vi "InfluxDriver.vi"(6 "body":string, 7 "dbwrite":string, 8 "error in (no error)":errorcluster, 9 "authorization":string, 10 "remote port":u16=8086, 11 "InfluxDB Address":string="128.8.27.25") -> (0 "error out":errorcluster, 2 "data out":string)   [LabVIEW 2013, in "ovenCtrl.lvlib"]
uses:
  ovenCtrl.lvlib
panel:
  out "concatenated string":string
  out "bytes written":i32
  # "Outputs"
  # "Inputs"
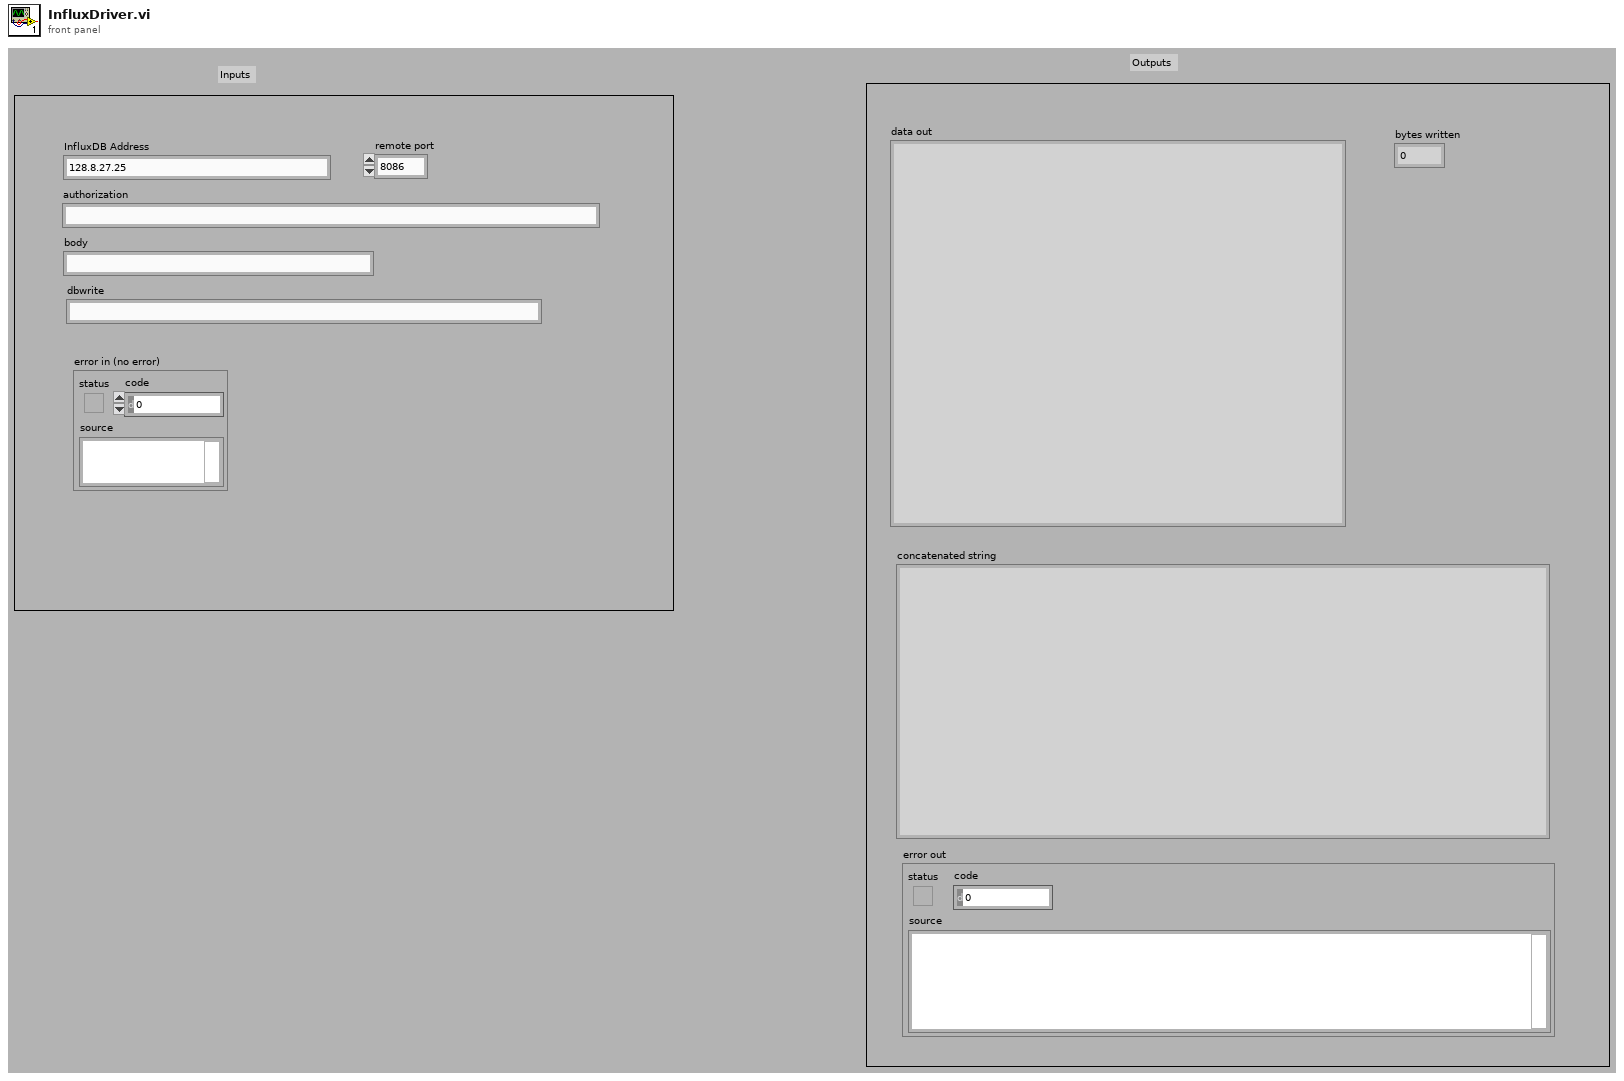
[diagram p1: front panel]
types:
  T1 = enum16{"Standard", "Buffered", "CRLF", "Immediate"}
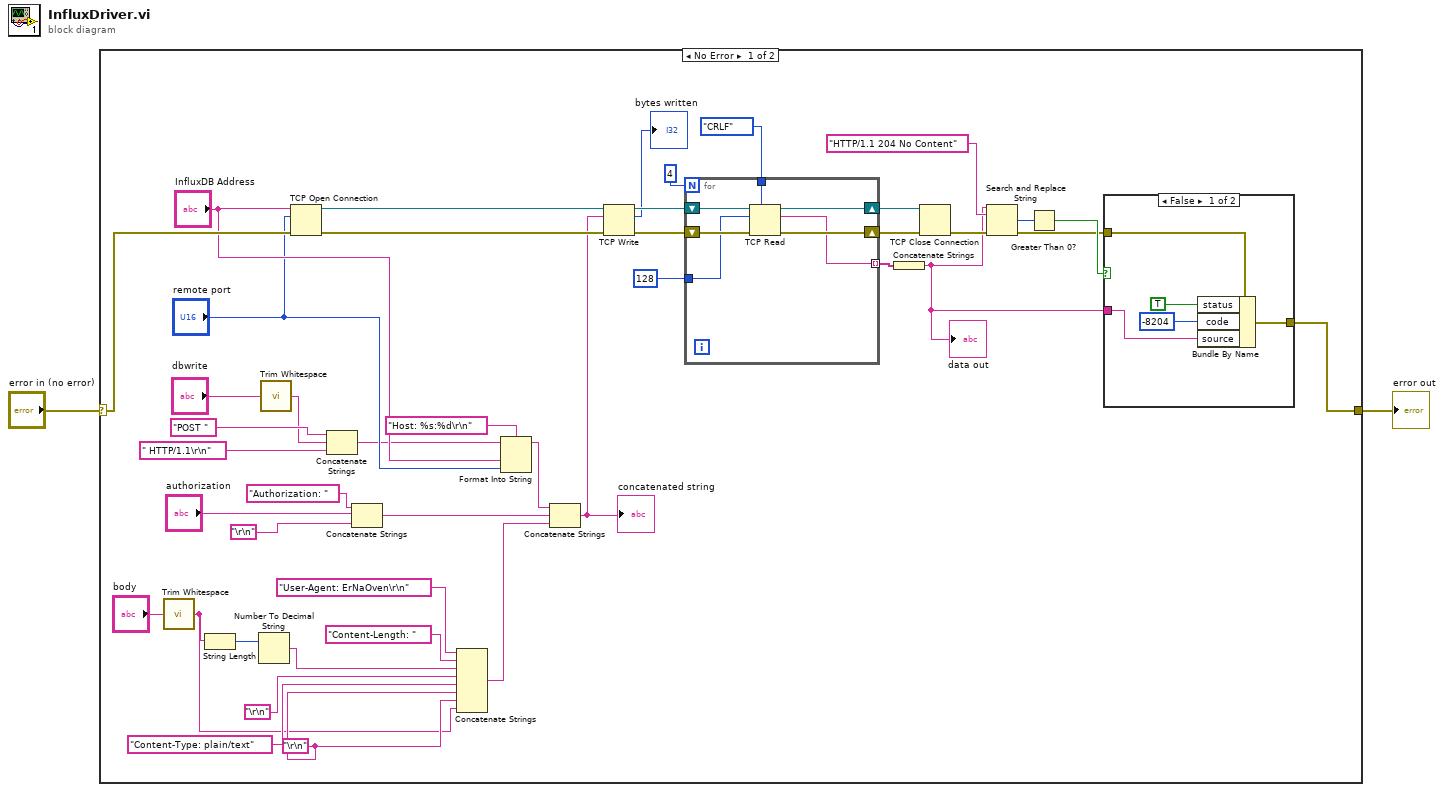
[diagram p0: block diagram]
diagram:
  n1 = case shown="No Error" "error in (no error)" {
    selector: "error in (no error)" -> [w13 w59]
    tunnel: [w12 w59] -> w1
    frame No Error {
      w27 = "\r\n"
      n2 = call <vilib>:"Trim Whitespace.vi"("string"="body") -> ("trimmed string"=w19:string)  [unwired: 1 in]
      n3 = String Length(string=w19) -> (length=w28:i32)
      n4 = Number To Decimal String(number=w28) -> (decimal integer string=w29:string)  [unwired: 1 in]
      n5 = call <vilib>:"Trim Whitespace.vi"("string"="dbwrite") -> ("trimmed string"=w22:string)  [unwired: 1 in]
      n6 = TCP Open Connection(address="InfluxDB Address", remote port or service name="remote port", error in (no error)=w13) -> (connection ID=w44:refnum<k5>, error out=w45:errorcluster)  [unwired: 2 in]
      n7 = Concatenate Strings("POST ", w22, " HTTP/1.1\r\n") -> (w5:string)
      n8 = Concatenate Strings("Authorization: ", "authorization", "\r\n") -> (w25:string)
      n9 = Concatenate Strings("User-Agent: ErNaOven\r\n" ("string"), "Content-Length: ", w29, "\r\n", "Content-Type: plain/text", w27, w27, w19) -> (w24:string)
      n10 = Format Into String(format string="Host: %s:%d\r\n", initial string=w5, "InfluxDB Address", "remote port") -> (resulting string=w4:string)  [unwired: 1 in, 1 out]
      n11 = Concatenate Strings(w4, w25, w24) -> (w21:string)
      "concatenated string" <- w21
      n12 = TCP Write(connection ID=w44, data in=w21, error in (no error)=w45) -> (connection ID out=w43:refnum<k5>, bytes written=→"bytes written":i32, error out=w42:errorcluster)  [unwired: 1 in]
      n13 = for {
        N: 4 -> [_]
        tunnel: 128 ("bytes to read") -> [w48]
        tunnel: T1."CRLF" ("mode (standard)") -> [w47]
        tunnel: [w46] -> w11 mode=indexing
        shift-right: [w49] -> w40
        shift-left: w43 -> [w52]
        shift-right: [w50] -> w41
        shift-left: w42 -> [w51]
        n14 = TCP Read(connection ID=w52, bytes to read=w48, error in (no error)=w51, 7:w47) -> (connection ID out=w49:refnum<k5>, data out=w46:string, error out=w50:errorcluster)  [unwired: 1 in]
      }
      n15 = Concatenate Strings(w11) -> (w10:string)
      "data out" <- w10
      n16 = TCP Close Connection(connection ID=w40, error in (no error)=w41) -> (error out=w18:errorcluster)  [unwired: 1 in, 1 out]
      n17 = Search and Replace String(input string=w10, search string="HTTP/1.1 204 No Content", error in=w18) -> (number of replacements=w16:i32, error out=w14:errorcluster)  [unwired: 5 in, 2 out]
      n18 = Greater Than 0?(x=w16) -> (x > 0?=w15:bool)
      n19 = case shown="False" w15 {
        tunnel: w10 -> [w54 _]
        tunnel: [w57 w58] -> w12
        tunnel: w14 -> [w56 w58]
        frame False {
          n20 = Bundle By Name(cluster=w56, "status"=TRUE, "code"=-8204, "source"=w54) -> (w57:errorcluster)
        }
        frame True {
        }
      }
    }
    frame Error {
    }
  }
  "error out" <- w1
